vi "1A Helper - LatLong to UTM.vi"(1 "East/West":string="N/A", 2 "Longitude":dbl, 3 "North/South":string="N/A", 4 "Latitude":dbl) -> (0 "Robot UTM Location":T1)   [LabVIEW 2011]
uses:
  2-Think/2 Typedefs/UTM Location.ctl
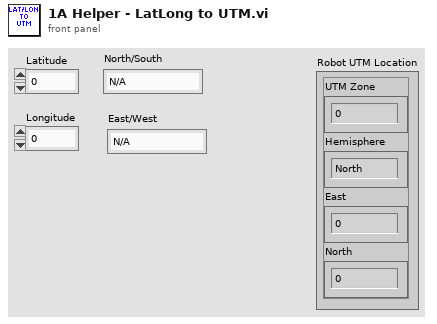
[diagram p1: front panel]
types:
  T1 = typedef "UTM Location.ctl" = cluster{"UTM Zone":dbl, "Hemisphere":enum16{"North", "South"}, "East":dbl, "North":dbl}
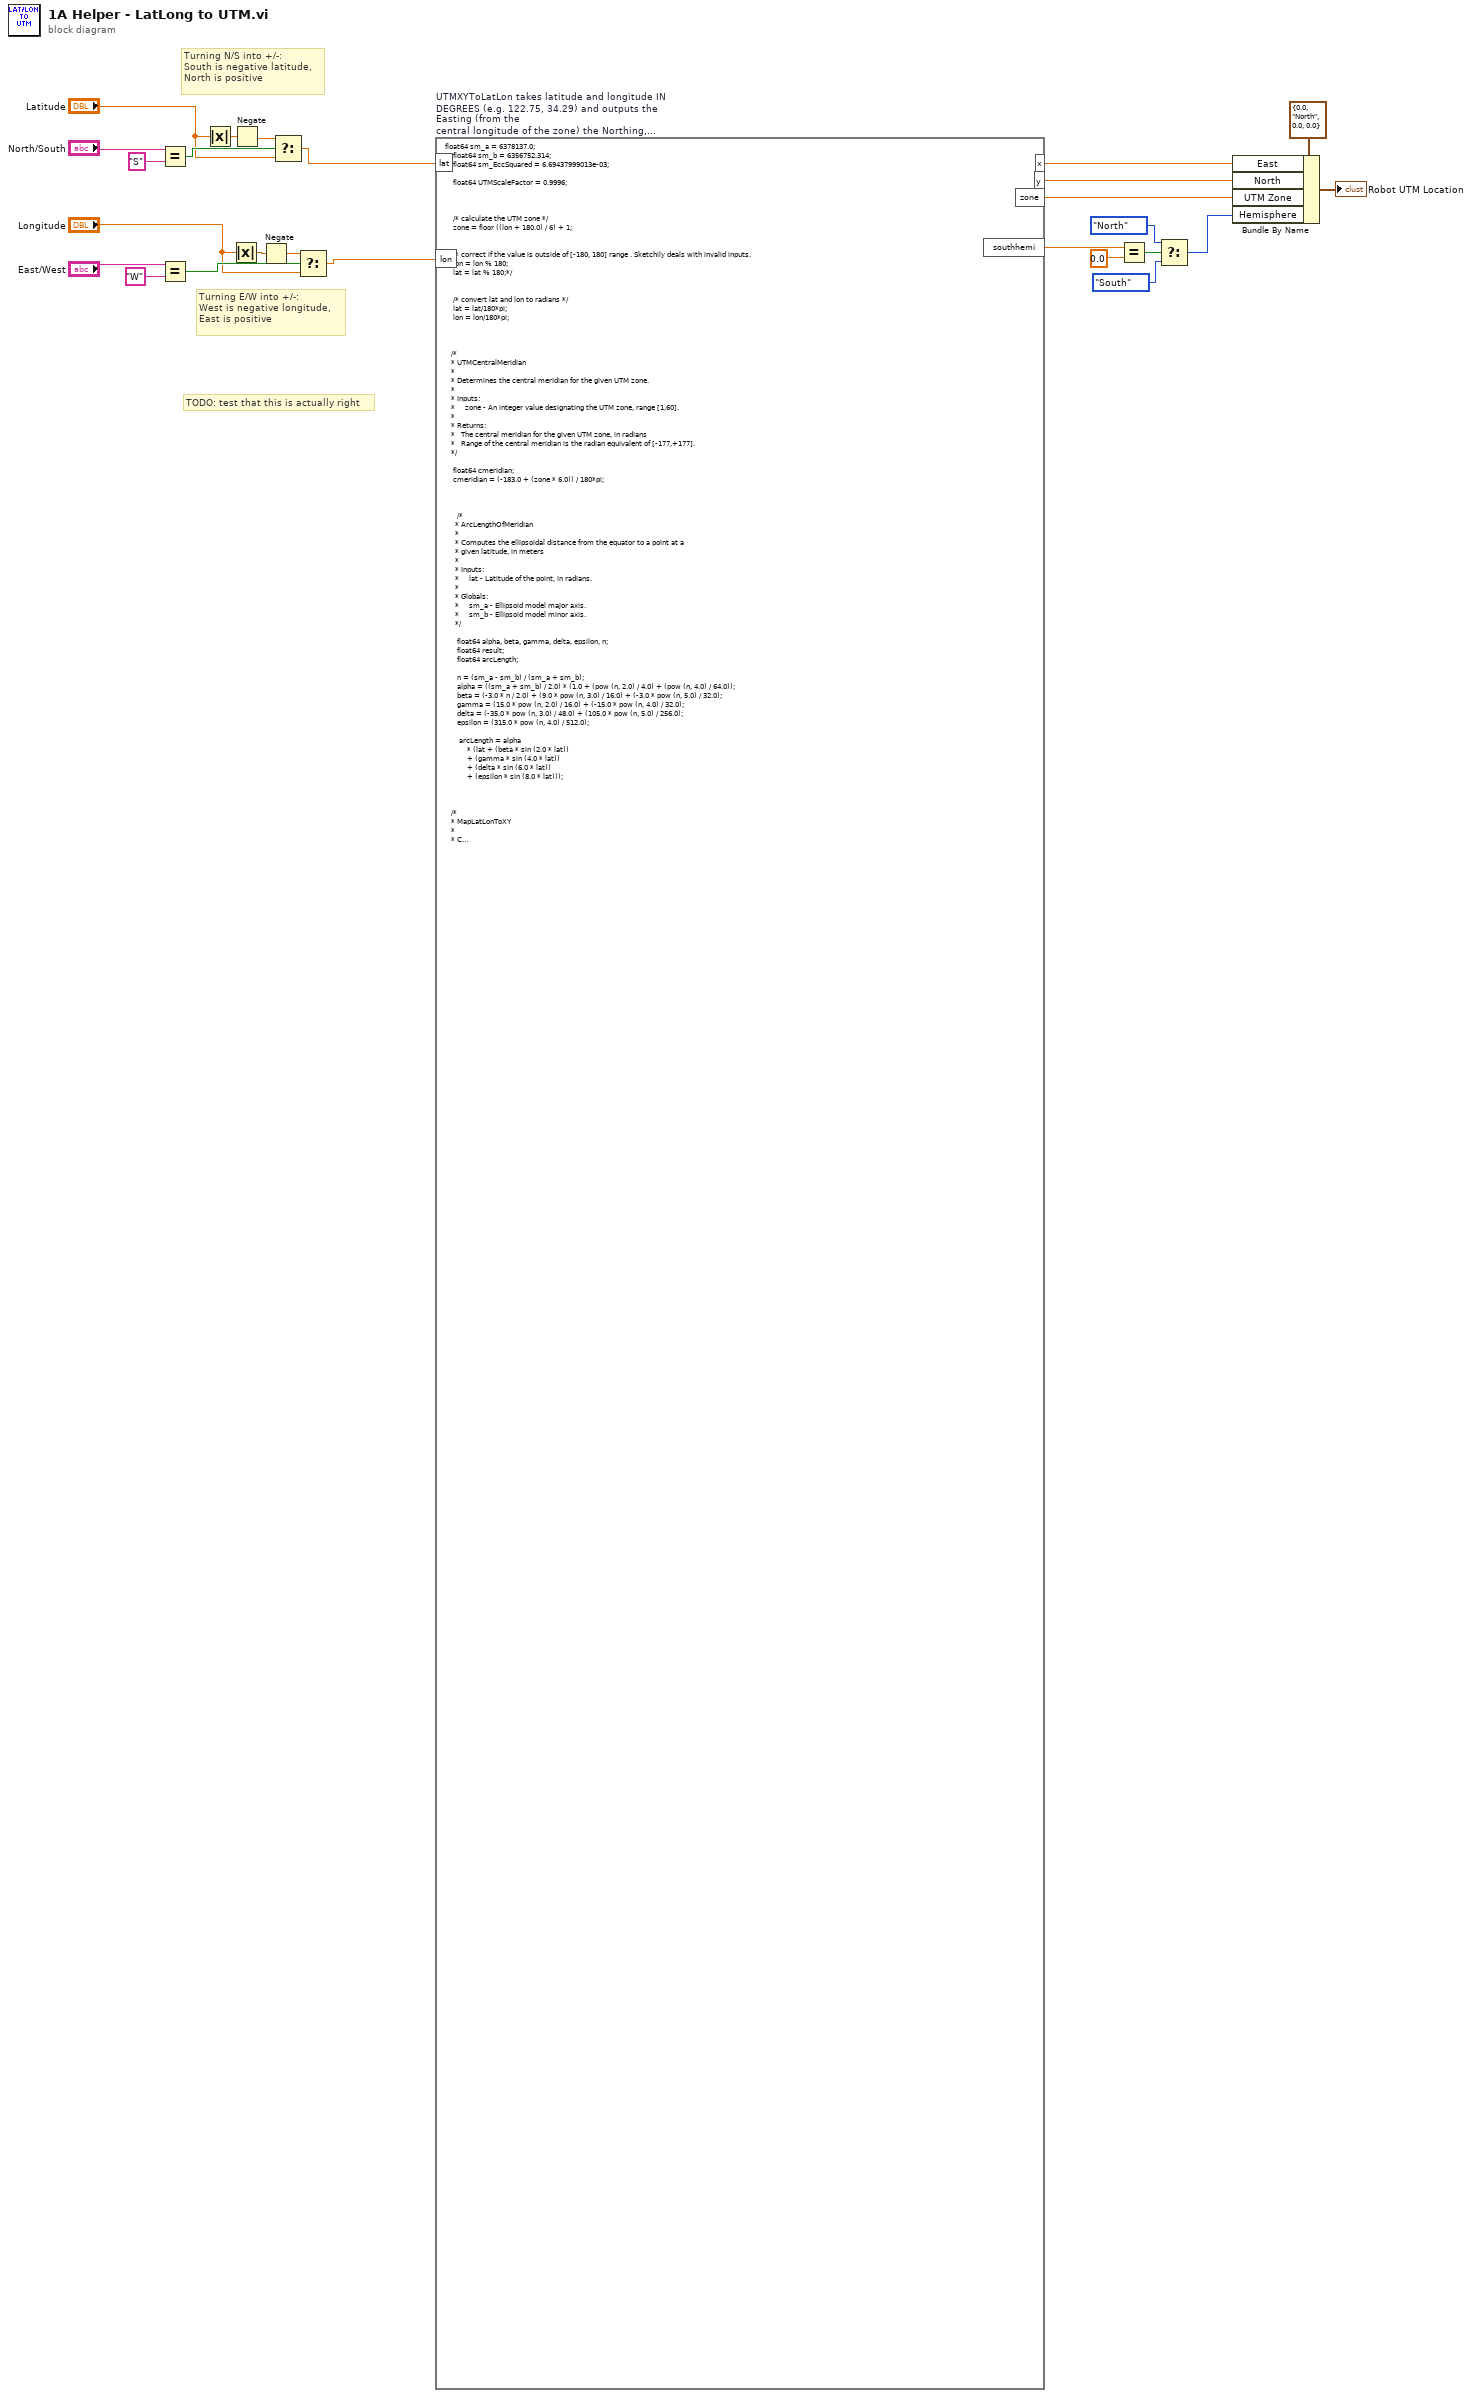
[diagram p0: block diagram]
diagram:
  # "Turning E/W into +/-:\nWest is negative longitude, \nEast is positive"
  # "Turning N/S into +/-:\nSouth is negative latitude, \nNorth is positive"
  # "TODO: test that this is actually right"
  n1 = Equal?(x="North/South", y="S" ("submatch 2")) -> (x = y?=w18:bool)
  n2 = Equal?(x="East/West", y="W" ("submatch 2")) -> (x = y?=w14:bool)
  n3 = Absolute Value(x="Latitude") -> (abs(x)=w9:dbl)
  n4 = Absolute Value(x="Longitude") -> (abs(x)=w8:dbl)
  n5 = Negate(x=w9) -> (-x=w17:dbl)
  n6 = Negate(x=w8) -> (-x=w15:dbl)
  n7 = Select(t=w17, s=w18, f="Latitude") -> (s? t:f=w16:dbl)
  n8 = Select(t=w15, s=w14, f="Longitude") -> (s? t:f=w12:dbl)
  n9 = formula code="float64 sm_a = 6378137.0;\n    float64 sm_b = 6356752.314;\n    float64 sm_EccSquared = 6.69437999013e-03;\n\n    float64 UTMScaleFactor = 0.9996;\n\n\n\n    /* calculate the UTM zone */\n    zone = floor ((lon + 180.0) / 6) + 1;\n\n\n    /* correct if the value is outside of [-180, 180] range . Sketchily deals with invalid inputs.\n    lon = lon % 180;\n    lat = lat % 180;*/\n\n\n    /* convert lat and lon to radians */\n    lat = lat/180*pi;\n    lon = lon/180*pi;\n\n\n\n\t\t /*\n\t\t\t* UTMCentralMeridian\n\t\t\t*\n\t\t\t* Determines the central meridian for the given UTM zone.\n\t\t\t*\n\t\t\t* Inputs:\n\t\t\t*     zone - An integer value designating the UTM zone, range [1,60].\n\t\t\t*\n\t\t\t* Returns:\n\t\t\t*   The central meridian for the given UTM zone, in radians\n\t\t\t*   Range of the central meridian is the radian equivalent of [-177,+177].\n\t\t\t*/\n\n\t\t\t\tfloat64 cmeridian;\n\t\t\t\tcmeridian = (-183.0 + (zone * 6.0)) / 180*pi;\n\t\t\n\n\n\t\t\t\t  /*\n\t\t\t\t\t* ArcLengthOfMeridian\n\t\t\t\t\t*\n\t\t\t\t\t* Computes the ellipsoidal distance from the equator to a point at a\n\t\t\t\t\t* given latitude, in meters\n\t\t\t\t\t*\n\t\t\t\t\t* Inputs:\n\t\t\t\t\t*     lat - Latitude of the point, in radians.\n\t\t\t\t\t*\n\t\t\t\t\t* Globals:\n\t\t\t\t\t*     sm_a - Ellipsoid model major axis.\n\t\t\t\t\t*     sm_b - Ellipsoid model minor axis.\n\t\t\t\t\t*/\n\n\t\t\t\t\t\tfloat64 alpha, beta, gamma, delta, epsilon, n;\n\t\t\t\t\t\tfloat64 result;\n      float64 arcLength;\n\n\t\t\t\t\t\tn = (sm_a - sm_b) / (sm_a + sm_b);\n\t\t\t\t\t\talpha = ((sm_a + sm_b) / 2.0) * (1.0 + (pow (n, 2.0) / 4.0) + (pow (n, 4.0) / 64.0));\n\t\t\t\t\t\tbeta = (-3.0 * n / 2.0) + (9.0 * pow (n, 3.0) / 16.0) + (-3.0 * pow (n, 5.0) / 32.0);\n\t\t\t\t\t\tgamma = (15.0 * pow (n, 2.0) / 16.0) + (-15.0 * pow (n, 4.0) / 32.0);\n\t\t\t\t\t\tdelta = (-35.0 * pow (n, 3.0) / 48.0) + (105.0 * pow (n, 5.0) / 256.0);\n\t\t\t\t\t\tepsilon = (315.0 * pow (n, 4.0) / 512.0);\n\t\t\t\t\t\n\t\t\t\t\t  arcLength = alpha\n\t\t\t\t\t\t     * (lat + (beta * sin (2.0 * lat))\n    \t\t\t\t\t\t\t+ (gamma * sin (4.0 * lat))\n\t\t\t\t    \t\t\t+ (delta * sin (6.0 * lat))\n\t\t\t\t\t\t\t    + (epsilon * sin (8.0 * lat)));\n\n\n\n\t\t\t/*\n\t\t\t* MapLatLonToXY\n\t\t\t*\n\t\t\t* Converts a latitude/longitude pair to x and y coordinates in the\n\t\t\t* Transverse Mercator projection. Transverse Mercator is not UTM until scaled\n\t\t\t* Inputs:\n   *\n\t\t\t*    lat - Latitude of the point, in radians.\n\t\t\t*    lon - Longitude of the point, in radians.\n\t\t\t*    cmeridian - Longitude of the central meridian to be used, in radians.\n\t\t\t*/\n\n\n\t\t\t\tfloat64 N, nu2, ep2, t, t2, l;\n\t\t\t\tfloat64 l3coef, l4coef, l5coef, l6coef, l7coef, l8coef;\n\t\t\t\tfloat64 tmp;\n\n\n\t\t\t\tep2 = (pow (sm_a, 2.0) - pow (sm_b, 2.0)) / pow (sm_b, 2.0);\n\t\t\t\tnu2 = ep2 * pow (cos (lat), 2.0);\n\t\t\t\tN = pow (sm_a, 2.0) / (sm_b * sqrt (1 + nu2));\n\n\t\t\t\tt = tan (lat);\n\t\t\t\tt2 = t * t;\n\t\t\t\ttmp = (t2 * t2 * t2) - pow (t, 6.0);\n\n\t\t\t\tl = lon - cmeridian;\n\n\t\t\t\t/* Precalculate coefficients for l**n in the equations below\n\t\t\t\t   so a normal human being can read the expressions for easting\n\t\t\t\t   and northing*/\n\n\n\t\t\t\tl3coef = 1.0 - t2 + nu2;\n\t\t\t\tl4coef = 5.0 - t2 + 9 * nu2 + 4.0 * (nu2 * nu2);\n\t\t\t\tl5coef = 5.0 - 18.0 * t2 + (t2 * t2) + 14.0 * nu2 - 58.0 * t2 * nu2;\n\t\t\t\tl6coef = 61.0 - 58.0 * t2 + (t2 * t2) + 270.0 * nu2 - 330.0 * t2 * nu2;\n\t\t\t\tl7coef = 61.0 - 479.0 * t2 + 179.0 * (t2 * t2) - (t2 * t2 * t2);\n\t\t\t\tl8coef = 1385.0 - 3111.0 * t2 + 543.0 * (t2 * t2) - (t2 * t2 * t2);\n\t\t\t\n\n\n\t\t\t\t/* Calculate easting (x) */\n\n  \t\t\tx = N * cos (lat) * l\n\t\t\t\t\t+ (N / 6.0 * pow (cos (lat), 3.0) * l3coef * pow (l, 3.0))\n\t\t\t\t\t+ (N / 120.0 * pow (cos (lat), 5.0) * l5coef * pow (l, 5.0))\n\t\t\t\t\t+ (N / 5040.0 * pow (cos (lat), 7.0) * l7coef * pow (l, 7.0));\t\t\t\n\n\n\n\t\t\t\t/* Calculate northing (y) */\n\t\t\t\t\n\t\t\t\ty = arcLength\n\t\t\t\t    + (t / 2.0 * N * pow (cos (lat), 2.0) * pow (l, 2.0))\n\t\t\t\t\t   + (t / 24.0 * N * pow (cos (lat), 4.0) * l4coef * pow (l, 4.0))\n\t\t\t\t\t   + (t / 720.0 * N * pow (cos (lat), 6.0) * l6coef * pow (l, 6.0))\n\t\t\t\t\t   + (t / 40320.0 * N * pow (cos (lat), 8.0) * l8coef * pow (l, 8.0));\n\t\n\n\n\t\n     /* Adjust easting and northing for UTM system. */\n     x = x * UTMScaleFactor + 500000.0;\n     y = y * UTMScaleFactor;\n     if (y < 0.0)\n         y = y + 10000000.0;\n\n\n\n     if (lat < 0)\n     southhemi = 1;\n     else\n     southhemi = 0;" "UTMXYToLatLon takes latitude and longitude IN DEGREES (e.g. 122.75, 34.29) and outputs the Easting (from the\ncentral longitude of the zone) the Northing, UTM zone and hemisphere. Equation is commented to some degree, but\nif you have questions talk to Eric Schneider"("lat"=w16, "lon"=w12) -> ("x"=w23:dbl, "y"=w21:dbl, "zone"=w22:dbl, "southhemi"=w6:dbl)
  n10 = Equal?(x=w6, y=0.0) -> (x = y?=w1:bool)
  n11 = Select(t=enum16{"North", "South"}."North" ("Hemisphere"), s=w1, f=enum16{"North", "South"}."South" ("Hemisphere")) -> (s? t:f=w3:enum16{"North", "South"})
  n12 = Bundle By Name(cluster=T1 {"UTM Zone"=0.0, "Hemisphere"=enum."North", "East"=0.0, "North"=0.0} ("Robot UTM Location"), "East"=w23, "North"=w21, "UTM Zone"=w22, "Hemisphere"=w3) -> (→"Robot UTM Location":T1)
